vi "test 2.vi"() -> ()   [LabVIEW 2012]
panel:
  out "Wz":dbl
  out "speed":dbl
  out "sign":i32
  out "b":i32
  out "a":dbl
  out "Degrees":dbl
  out "Angle":dbl
  in  "stop":bool
  in  "x":i32
  in  "y":i32
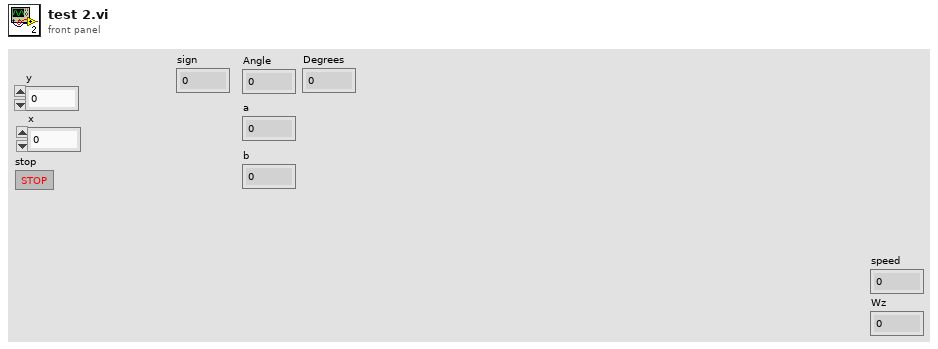
[diagram p1: front panel]
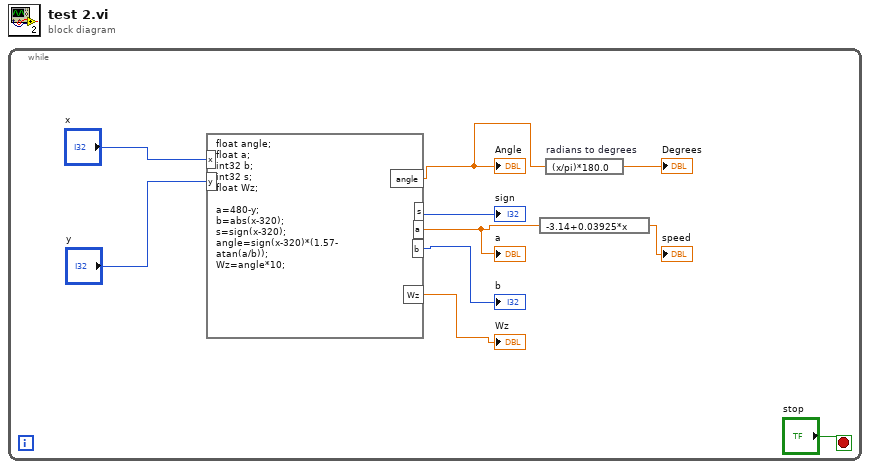
[diagram p0: block diagram]
diagram:
  n1 = while {
    stop <- "stop" stop-if-true
    n2 = formula code="float angle;\nfloat a;\nint32 b;\nint32 s;\nfloat Wz;\n\na=480-y;\nb=abs(x-320);\ns=sign(x-320);\nangle=sign(x-320)*(1.57-\natan(a/b));\nWz=angle*10;"("x"="x", "y"="y") -> ("angle"=w1:dbl, "a"=w4:dbl, "b"=→"b":i32, "s"=→"sign":i32, "Wz"=→"Wz":dbl)
    "Angle" <- w1
    "a" <- w4
    n3 = expression code="-3.14+0.03925*x"(w4) -> (→"speed":dbl)
    n4 = expression code="(x/pi)*180.0" "radians to degrees"(w1) -> (→"Degrees":dbl)
  }
